vi "Store Data.vi"(8 "Error In":errorcluster, 10 "LHW-DataCollection":refnum<class "LHW-DataCollection.lvclass">, 11 "LHW-Storage-Actor in":refnum<class "LHW-Storage-Actor.lvclass">) -> (0 "Error Out":errorcluster, 3 "LHW-Storage-Actor out":refnum<class "LHW-Storage-Actor.lvclass">)   [LabVIEW 2014, in "LHW-Storage.lvlib" / "LHW-Storage-Actor.lvclass"]
doc: "Store received data."
uses:
  LHW-Storage-Actor.lvclass
  Classes/LHW-Data/LHW-DataCollection/LHW-DataCollection.lvclass
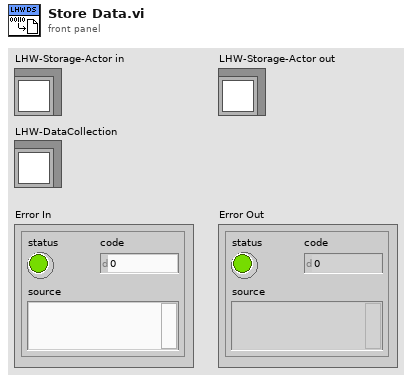
[diagram p1: front panel]
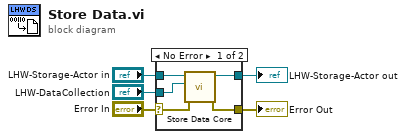
[diagram p0: block diagram]
diagram:
  n1 = case shown="No Error" "Error In" {
    selector: "Error In" -> [w8 w12]
    tunnel: [w7 w12] -> w4
    tunnel: [w9 w11] -> w2
    tunnel: "LHW-Storage-Actor in" -> [w10 w11]
    tunnel: "LHW-DataCollection" -> [w6 _]
    frame No Error {
      n2 = call-dynamic "Store Data Core.vi"("Error In"=w8, "LHW-DataCollection"=w6, "LHW-Storage-Actor in"=w10) -> ("Error Out"=w7:errorcluster, "LHW-Storage-Actor out"=w9:refnum<class "LHW-Storage-Actor.lvclass">)  [unwired: 7 in]
    }
    frame Error {
    }
  }
  "Error Out" <- w4
  "LHW-Storage-Actor out" <- w2
